vi "myRIO_BRig_RT_dataCurrent_IallReward_R.vi"() -> (2 "output_IallReward_R":i32)   [LabVIEW 2014]
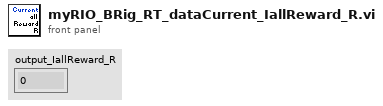
[diagram p1: front panel]
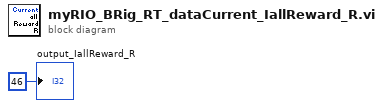
[diagram p0: block diagram]
diagram:
  "output_IallReward_R" <- 46 ("output_iBlock")
